vi "Initialize-queues.vi"(8 "error in (no error)":errorcluster, 9 "Batch size":i32, 10 "Image buffer size":i32, 11 "Buffers in":refnum<class "CV-Buffers.lvclass">) -> (0 "error out":errorcluster, 3 "Buffers out":refnum<class "CV-Buffers.lvclass">)   [LabVIEW 2013, in "CameraVision.lvlib" / "CV-Buffers.lvclass"]
uses:
  CV-Buffers.lvclass
  Mapping-buffer.ctl
  Temperature/Temperature-characteristics.ctl
  Analysis/Characteristics-cluster.ctl
  Processing-buffer.ctl
  <vilib>/vision/Image Controls.llb/IMAQ Image.ctl
  Storage-buffer.ctl
  CV-Buffers.lvclass/CV-Buffers.ctl
  Analysis/CV-Analysis.lvclass
  Temperature/CV-Temperature.lvclass
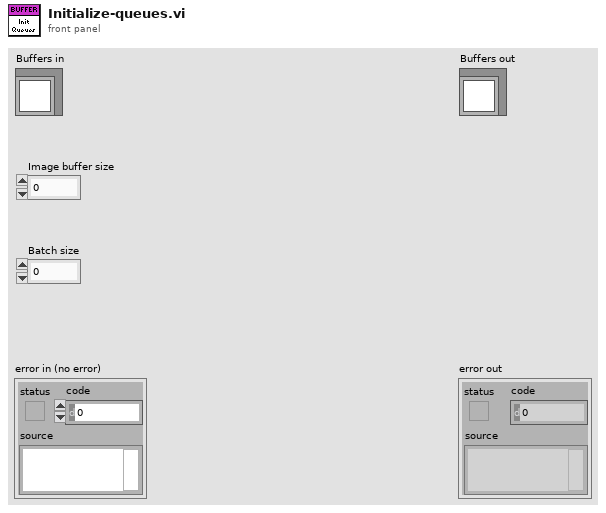
[diagram p1: front panel]
types:
  T1 = typedef "CameraVision.lvlib/CV-Buffers.lvclass/Storage-buffer.ctl" = cluster{"Index":i32, "Time":timestamp, "Raw images":T2[], "Corrected images":T2[], "Binary images":T2[], "Temperature characteristics":T3, "Characteristics":T4[], "Temperature field":dbl[][]}
  T2 = typedef "IMAQ Image.ctl" = refnum<image>
  T3 = typedef "CameraVision.lvlib/CV-Temperature.lvclass/Temperature-characteristics.ctl" = cluster{"Average temperature ":dbl, "Max. temperature":dbl, "Min. temperature":dbl, "Stand. dev. temperature":dbl, "Datapoints":dbl}
  T4 = typedef "CameraVision.lvlib/CV-Analysis.lvclass/Characteristics-cluster.ctl" = cluster{"Average intensity":dbl, "Peak intensity":dbl, "Melt-pool size":dbl, "Melt-pool aspect ratio":dbl, "Melt-pool fragments":dbl, "Centre of mass X":dbl, "Centre of mass Y":dbl, "Orientation":dbl}
  T5 = typedef "CameraVision.lvlib/CV-Buffers.lvclass/Processing-buffer.ctl" = cluster{"Index":i32, "Time":timestamp, "Raw images":T2[]}
  T6 = typedef "CameraVision.lvlib/CV-Buffers.lvclass/Mapping-buffer.ctl" = cluster{"Time":timestamp, "Index":i32, "Temperature characteristics":T3, "Characteristics":T4[], "Xcoord":sgl, "Ycoord":sgl}
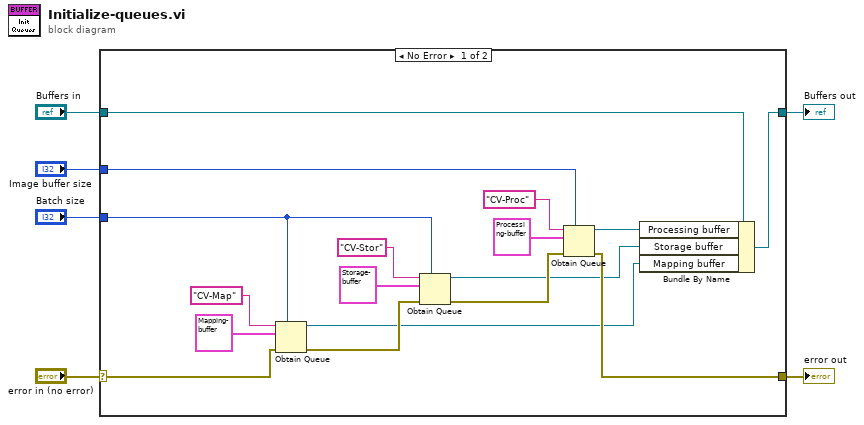
[diagram p0: block diagram]
diagram:
  n1 = case shown="No Error" "error in (no error)" {
    selector: "error in (no error)" -> [w12 w25]
    tunnel: [w11 w25] -> w5
    tunnel: [w10 w24] -> w3
    tunnel: "Buffers in" -> [w23 w24]
    tunnel: "Batch size" -> [w18 _]
    tunnel: "Image buffer size" -> [w19 _]
    frame No Error {
      n2 = Obtain Queue(max queue size (-1, unlimited)=w18, name (unnamed)="CV-Map", element data type=T6 {"Time"=timestamp(0 s since 1904-01-01), "Index"=0, "Temperature characteristics"={"Average temperature "=0.0, "Max. temperature"=0.0, "Min. temperature"=0.0, "Stand. dev. temperature"=0.0, "Datapoints"=0.0}, "Characteristics"=[], "Xcoord"=0.0, "Ycoord"=0.0} ("Mapping element"), error in (no error)=w12) -> (queue out=w7:refnum<queue>, error out=w14:errorcluster)  [unwired: 1 in, 1 out]
      n3 = Obtain Queue(max queue size (-1, unlimited)=w18, name (unnamed)="CV-Stor", element data type=T1 {"Index"=0, "Time"=timestamp(0 s since 1904-01-01), "Raw images"=[], "Corrected images"=[], "Binary images"=[], "Temperature characteristics"={"Average temperature "=0.0, "Max. temperature"=0.0, "Min. temperature"=0.0, "Stand. dev. temperature"=0.0, "Datapoints"=0.0}, "Characteristics"=[], "Temperature field"=[]} ("Storage element"), error in (no error)=w14) -> (queue out=w8:refnum<queue>, error out=w13:errorcluster)  [unwired: 1 in, 1 out]
      n4 = Obtain Queue(max queue size (-1, unlimited)=w19, name (unnamed)="CV-Proc", element data type=T5 {"Index"=0, "Time"=timestamp(0 s since 1904-01-01), "Raw images"=[]} ("Processing element"), error in (no error)=w13) -> (queue out=w9:refnum<queue>, error out=w11:errorcluster)  [unwired: 1 in, 1 out]
      n5 = Bundle By Name(cluster=w23, "Processing buffer"=w9, "Storage buffer"=w8, "Mapping buffer"=w7) -> (w10:refnum<class "CV-Buffers.lvclass">)
    }
    frame Error {
    }
  }
  "error out" <- w5
  "Buffers out" <- w3
